vi "Do.vi"(8 "error in (no error)":errorcluster, 10 "Actor in":refnum<class "Actor.lvclass">, 11 "Device Init CVT MSG":refnum<class "Device Init CVT MSG.lvclass">) -> (0 "error out":errorcluster, 2 "Actor out":refnum<class "Actor.lvclass">)   [LabVIEW 2014, in "Controller.lvlib" / "Device Init CVT MSG.lvclass"]
doc: "(<B>Filename</B>: Actor Framework.lvlib:Message.lvclass:Do.vi)\n\nDefines what a message does when it is received by an actor. Generally, a message instructs an actor to invoke one of its methods. By default, this method does nothing. A child class must override it to define behavior. Create a child class by using the Actor Framework Message Maker dialog box."
uses:
  Device Init CVT MSG.lvclass
  <vilib>/ActorFramework/Actor/Actor.lvclass
  Controller.lvclass
  reusable/DAQ Device/Messages/Generic CVT Init/Generic Init CVT Message.lvclass/Generic Init CVT Message.ctl
  SuperActor/Ex Nested.lvclass/Ex Nested.ctl
  reusable/DAQ Device/Messages/Generic CVT Init/Read DevID.vi
  reusable/DAQ Device/Messages/Generic CVT Init/Read SP.vi
  SuperActor/Read CVT Session.vi
  <userlib>/_Session Fwk/Session - Root.lvclass
  reusable/Session APIs/CVT/CVT.lvclass
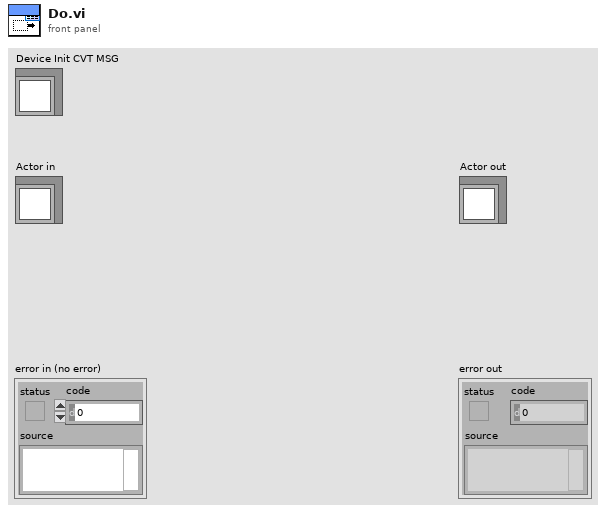
[diagram p1: front panel]
types:
  T1 = typedef "Session - Root.lvclass/Session Handle.ctl" = refnum<data-value>
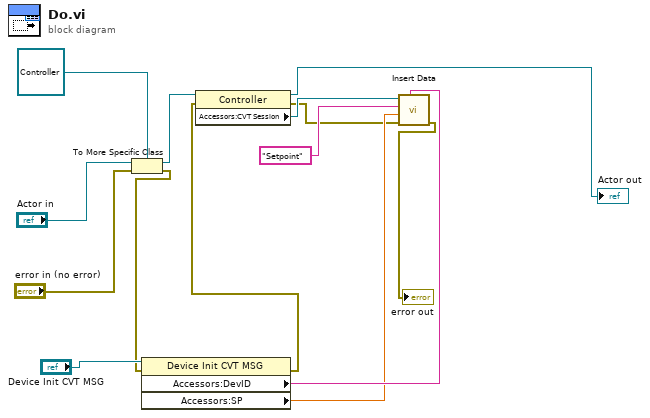
[diagram p0: block diagram]
diagram:
  n1 = To More Specific Class(target class=refnum<class "Controller.lvclass"> refnum ("Controller.lvlib:Controller"), reference="Actor in", error in="error in (no error)") -> (specific class reference=w9:refnum<class "Controller.lvclass">, error out=w10:errorcluster)
  n2 = property class="Device Init CVT MSG"(reference="Device Init CVT MSG", error in=w10) -> (error out=w4:errorcluster, "Accessors:DevID"=w7:string, "Accessors:SP"=w5:dbl)  [unwired: 1 out]
  n3 = property class="Controller"(reference=w9, error in=w4) -> (reference out=→"Actor out":refnum<class "Controller.lvclass">, error out=w3:errorcluster, "Accessors:CVT Session"=w8:T1)
  n4 = call "Insert Data.vi"("tag"=w7, "error in"=w3, "Data"=w5, "Group"="Setpoint" ("tag"), "CVT Session In"=w8) -> ("error out"=→"error out":errorcluster)  [unwired: 5 in, 1 out]
